vi "startOpenLoopScan.vi"(8 "error in (no error)":errorcluster, 11 "Context in":refnum<class "Context.lvclass">) -> (0 "error out":errorcluster, 3 "Context out":refnum<class "Context.lvclass">)   [LabVIEW 2015, in "Context.lvclass"]
uses:
  Context.lvclass
  Context.lvclass/Context.ctl
  State/State.lvclass
  Model/Model/Model.lvclass
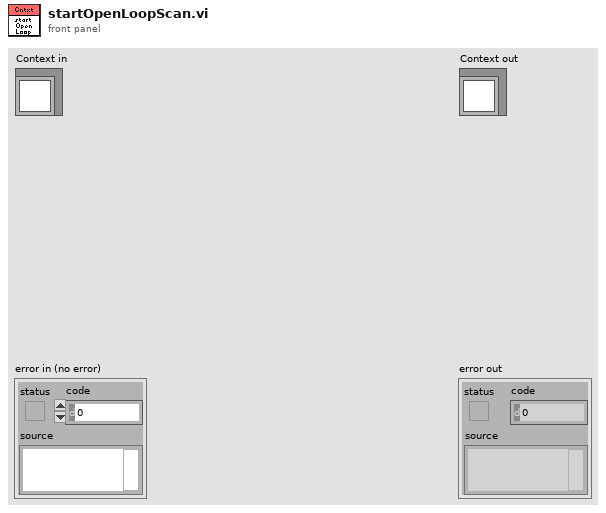
[diagram p1: front panel]
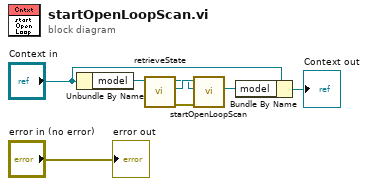
[diagram p0: block diagram]
diagram:
  n1 = Unbundle By Name("Context in") -> ("model"=w7:refnum<class "Model.lvclass">)
  n2 = call "retrieveState.vi"("Model in"=w7) -> ("error out"=w1:errorcluster, "state"=w3:refnum<class "State.lvclass">, "Model out"=w2:refnum<class "Model.lvclass">)  [unwired: 8 in]
  n3 = call-dynamic "startOpenLoopScan.vi"("error in (no error)"=w1, "model"=w2, "State in"=w3) -> ("model 2"=w4:refnum<class "Model.lvclass">)  [unwired: 6 in, 2 out]
  n4 = Bundle By Name(cluster="Context in", "model"=w4) -> (→"Context out":refnum<class "Context.lvclass">)
  "error out" <- "error in (no error)"
